vi "Add ECAT Slave from Config.vi"(8 "error in (no error)":errorcluster, 10 "Section Ptr":T4 format="%.0x", 11 "Slave":T1) -> (0 "error out":errorcluster)   [LabVIEW 2019, in "SEECD System Explorer.lvlib"]
uses:
  SEECD System Explorer.lvlib
  <vilib>/NI VeriStand/Custom Device API/Custom Device Item Ref.ctl
  Type Defs/Host - Slave.ctl
  Type Defs/Host - Module.ctl
  Type Defs/IOV Container Contents.ctl
  <vilib>/NI VeriStand/Custom Device API/Custom Device Channel.ctl
  <vilib>/NI VeriStand/Custom Device API/Custom Device Channel Type.ctl
  Includes/Modules.lvlibp/RSI Module/Slot Settings.ctl
  Includes/Modules.lvlibp/RSI Module/Module Models.ctl
  Shared/Globals/Scan Engine GUIDs.vi
  Shared/Globals/String Constants.vi
  Shared/Globals/Property Strings.vi
  <vilib>/NI VeriStand/Custom Device API/Set Item Property (String).vi
  Includes/Modules.lvlibp/RSI Module/Class Property Strings.vi
  Includes/Modules.lvlibp/RemIO Module/RemIO Module.lvclass
  Includes/Modules.lvlibp/RSI Module/RSI Module.lvclass
  <vilib>/NI VeriStand/Custom Device API/Custom Device API.lvlib
  Shared/SEECD Shared.lvlib
  Includes/Modules.lvlibp
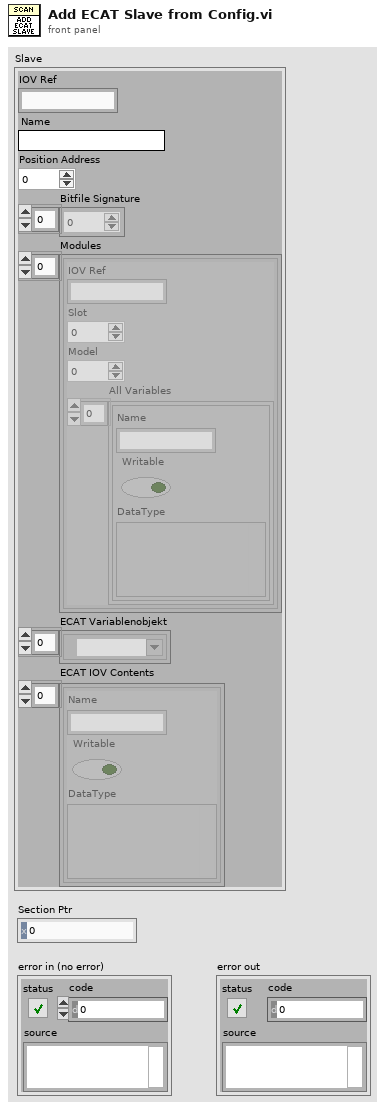
[diagram p1: front panel]
types:
  T1 = typedef "SEECD System Explorer.lvlib/Host - Slave.ctl" = cluster{"IOV Ref":string, "Name":string, "Position Address":u16, "Bitfile Signature":u8[], "Modules":T2[], "ECAT Variablenobjekt":refnum<k21>[], "ECAT IOV Contents":T3[]}
  T2 = typedef "SEECD System Explorer.lvlib/Host - Module.ctl" = cluster{"IOV Ref":string, "Slot":u32, "Model":u32, "All Variables":T3[]}
  T3 = typedef "SEECD System Explorer.lvlib/IOV Container Contents.ctl" = cluster{"Name":string, "Writable":bool, "DataType":variant}
  T4 = typedef "Custom Device API.lvlib/Custom Device Item Ref.ctl" = u64
  T5 = typedef "Custom Device API.lvlib/Custom Device Channel Type.ctl" = enum16{"Input", "Output"}
  T6 = typedef "Modules.lvlibp/RSI Module.lvclass/Slot Settings.ctl" = cluster{"Slot":u32, "EtherCAT?":bool}
  T7 = typedef "Modules.lvlibp/RSI Module.lvclass/Module Models.ctl" = enum16{"Empty", "NI 9201", "NI 9203", "NI 9205", "NI 9206", "NI 9207", "NI 9208", "NI 9209", "NI 9210", "NI 9211", "NI 9212", "NI 9213", "NI 9214", "NI 9215", "NI 9216", "NI 9217", "NI 9219", "NI 9220", "NI 9221", "NI 9222", "NI 9223", "NI 9224", "NI 9225", "NI 9226", "NI 9227", "NI 9228", "NI 9229", "NI 9233", "NI 9234", "NI 9235", "NI 9236", "NI 9237", "NI 9239", "NI 9242", "NI 9244", "NI 9253", "NI 9263", "NI 9264", "NI 9265", "NI 9266", "NI 9269", "NI 9344", "NI 9350", "NI 9375", "NI 9401", "NI 9402", "NI 9403", "NI 9411", "NI 9421", "NI 9422", "NI 9423", "NI 9425", "NI 9426", "NI 9435", "NI 9436", "NI 9437", "NI 9472", "NI 9474", "NI 9475", "NI 9476", "NI 9477", "NI 9478", "NI 9481", "NI 9482", "NI 9485"}
  T8 = typedef "Custom Device API.lvlib/Custom Device Channel.ctl" = cluster{"Type":T5, "Units":string, "Default Value":dbl, "Faultable":bool, "Scalable":bool}
  T9 = typedef "SEECD Shared.lvlib/ECAT Channel Data Type.ctl" = enum16{"Boolean", "Fixed Point", "Int8", "Int16", "Int32", "Int64", "U32 Bit Field", "UInt8", "UInt16", "UInt32", "UInt64", "Other", "DBL", "SGL"}
  T10 = typedef "Modules.lvlibp/Custom Device API.lvlib/Custom Device Item Ref.ctl" = u64
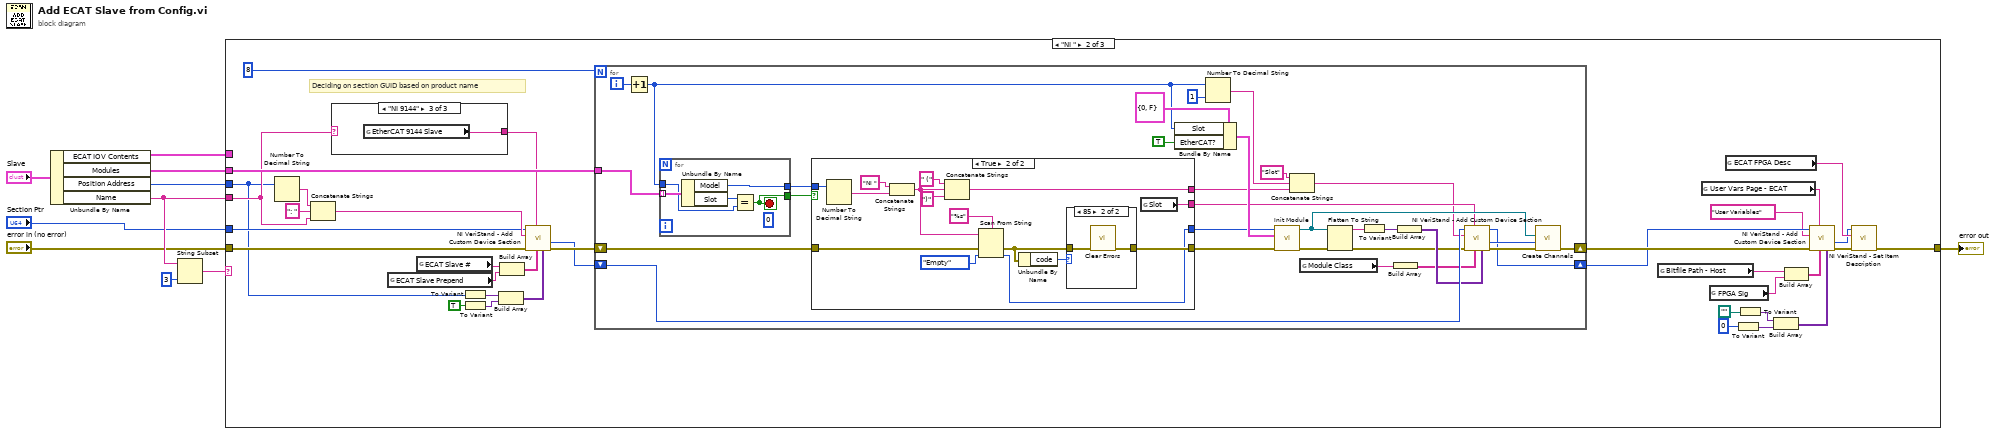
[diagram p0: block diagram]
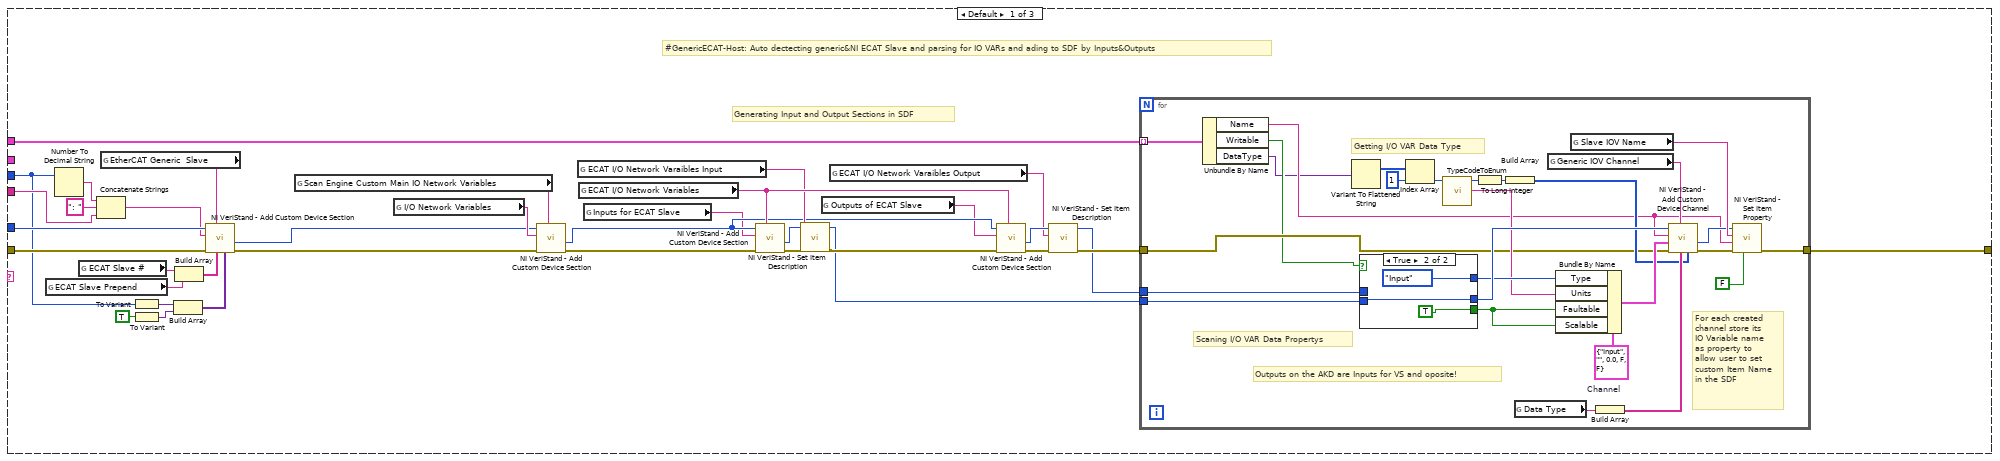
[diagram p2: hidden frame]
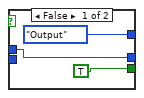
[diagram p3: hidden frame]
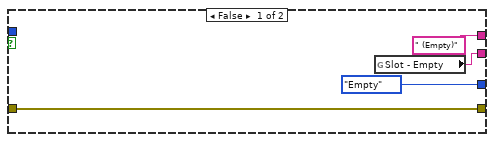
[diagram p4: hidden frame]
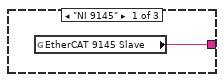
[diagram p6: hidden frame]
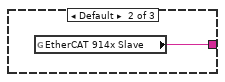
[diagram p7: hidden frame]
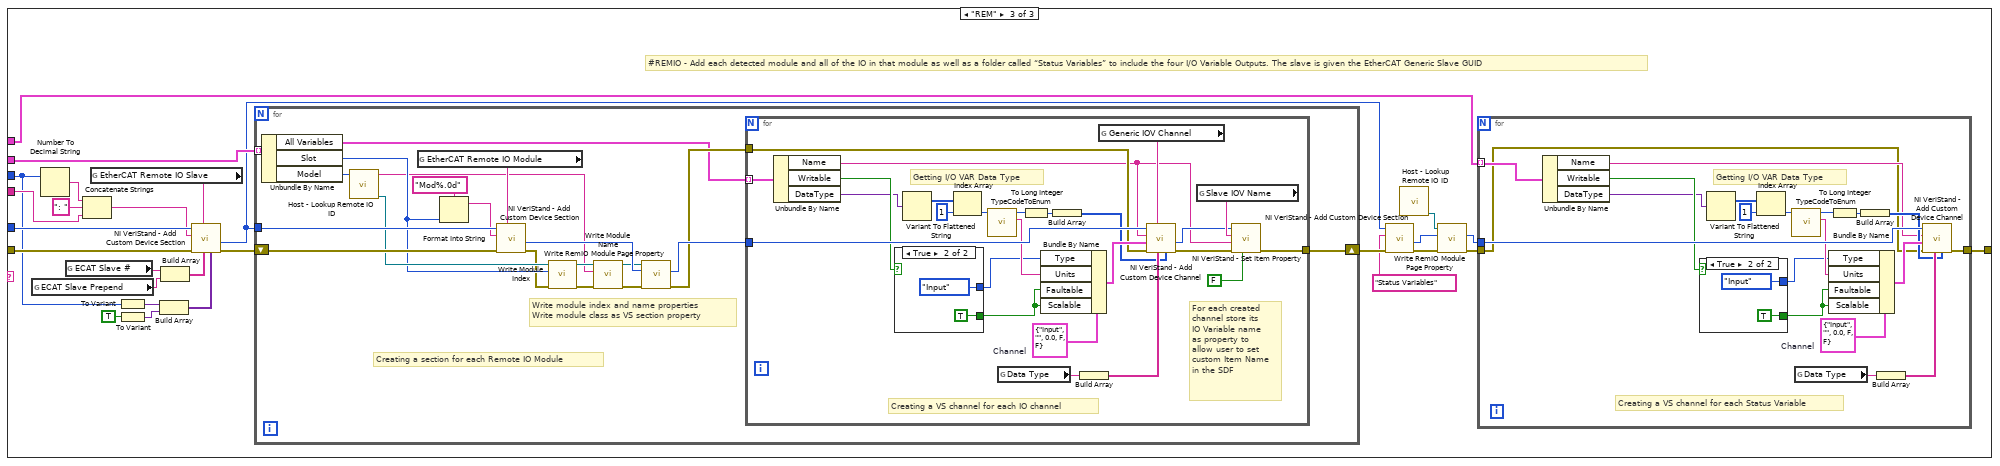
[diagram p8: hidden frame]
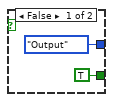
[diagram p9: hidden frame]
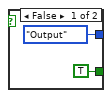
[diagram p10: hidden frame]
diagram:
  n1 = Unbundle By Name("Slave") -> ("ECAT IOV Contents"=w7:T3[], "Modules"=w4:T2[], "Position Address"=w9:u16, "Name"=w10:string)
  n2 = String Subset(string=w10, length (rest)=3 ("Länge (Rest)")) -> (substring=w8:string)  [unwired: 1 in]
  n3 = case shown="\"NI \"" w8 {
    tunnel: "error in (no error)" -> [w28 w98 w191]
    tunnel: w4 -> [_ w97 w200]
    tunnel: [w45 w96 w198] -> w5
    tunnel: w7 -> [w46 _ w197]
    tunnel: "Section Ptr" -> [w27 w83 w188]
    tunnel: w9 -> [w11 w80 w175]
    tunnel: w10 -> [w14 w82 w178]
    frame Default {
      # "#GenericECAT-Host: Auto dectecting generic&NI ECAT Slave and parsing for IO VARs and ading to SDF by Inputs&Outputs"
      # "Generating Input and Output Sections in SDF"
      n4 = global read "Property Strings.vi" "ECAT Slave Prepend"() -> (w18:string)
      n5 = Number To Decimal String(number=w11) -> (decimal integer string=w21:string)  [unwired: 1 in]
      n6 = global read "Property Strings.vi" "ECAT Slave #"() -> (w19:string)
      n7 = Concatenate Strings(w21, ": " ("string"), w14) -> (w23:string)
      n8 = global read "Scan Engine GUIDs.vi" "EtherCAT Generic  Slave"() -> (w24:string)
      n9 = To Variant(anything=w11) -> (Variant=w17:variant)
      n10 = To Variant(anything=TRUE) -> (Variant=w16:variant)
      n11 = Build Array(w17, w16) -> (w13:variant[])
      n12 = Build Array(w19, w18) -> (w20:string[])
      n13 = call <vilib>:"NI VeriStand - Add Custom Device Section.vi"("Property Values"=w13, "Property names"=w20, "GUID (Default Section)"=w24, "error in (no error)"=w28, "Section Name"=w23, "Parent Ref in"=w27) -> ("error out"=w25:errorcluster, "Section Ptr"=w26:T4)  [unwired: 2 in, 2 out]
      n14 = global read "Scan Engine GUIDs.vi" "Scan Engine Custom Main IO Network Variables"() -> (w38:string)
      n15 = global read "Property Strings.vi" "I/O Network Variables"() -> (w31:string)
      n16 = call <vilib>:"NI VeriStand - Add Custom Device Section.vi"("GUID (Default Section)"=w38, "error in (no error)"=w25, "Section Name"=w31, "Parent Ref in"=w26) -> ("error out"=w32:errorcluster, "Section Ptr"=w33:T4)  [unwired: 4 in, 2 out]
      n17 = global read "String Constants.vi" "ECAT I/O Network Varaibles Input"() -> (w34:string)
      n18 = global read "Scan Engine GUIDs.vi" "ECAT I/O Network Variables"() -> (w35:string)
      n19 = global read "Property Strings.vi" "Inputs for ECAT Slave"() -> (w30:string)
      n20 = call <vilib>:"NI VeriStand - Add Custom Device Section.vi"("GUID (Default Section)"=w35, "error in (no error)"=w32, "Section Name"=w30, "Parent Ref in"=w33) -> ("error out"=w44:errorcluster, "Section Ptr"=w37:T4)  [unwired: 4 in, 2 out]
      n21 = call <vilib>:"NI VeriStand - Set Item Description.vi"("error in (no error)"=w44, "Description"=w34, "Item Ref in"=w37) -> ("error out"=w43:errorcluster, "Item Ref out"=w42:T4)  [unwired: 6 in, 1 out]
      n22 = global read "Property Strings.vi" "Outputs of ECAT Slave"() -> (w29:string)
      n23 = global read "String Constants.vi" "ECAT I/O Network Varaibles Output"() -> (w12:string)
      n24 = call <vilib>:"NI VeriStand - Add Custom Device Section.vi"("GUID (Default Section)"=w35, "error in (no error)"=w43, "Section Name"=w29, "Parent Ref in"=w33) -> ("error out"=w41:errorcluster, "Section Ptr"=w36:T4)  [unwired: 4 in, 2 out]
      n25 = call <vilib>:"NI VeriStand - Set Item Description.vi"("error in (no error)"=w41, "Description"=w12, "Item Ref in"=w36) -> ("error out"=w40:errorcluster, "Item Ref out"=w39:T4)  [unwired: 6 in, 1 out]
      n26 = for {
        tunnel: w46 -> [w50] mode=indexing
        tunnel: [w55] -> w45
        tunnel: w40 -> [w51]
        tunnel: w39 -> [w68]
        tunnel: w42 -> [w66]
        w73 = T8 {"Type"=enum."Input", "Units"="", "Default Value"=0.0, "Faultable"=FALSE, "Scalable"=FALSE}  # Channel
        # "For each created channel store its IO Variable name as property to allow user to set custom Item Name in the SDF"
        # "Getting I/O VAR Data Type"
        # "Scaning I/O VAR Data Propertys"
        # "Outputs on the AKD are Inputs for VS and oposite!"
        n27 = Unbundle By Name(w50) -> ("Name"=w49:string, "Writable"=w48:bool, "DataType"=w47:variant)
        n28 = Variant To Flattened String(Variant=w47) -> (1:w70:i16[])  [unwired: 1 out]
        n29 = case shown="True" w48 {
          tunnel: [Custom_Device_Channel_Type."Output" ("Type") Custom_Device_Channel_Type."Input" ("Type")] -> w62
          tunnel: [w74 w77] -> w67
          tunnel: w68 -> [w74 _]
          tunnel: w66 -> [_ w77]
          tunnel: [TRUE TRUE] -> w65
          frame False {
          }
          frame True {
          }
        }
        n30 = Index Array(array=w70, index=1) -> (element=w60:i16)
        n31 = call "TypeCodeToEnum.vi"("Type Code (numbers in hexadecimal)"=w60) -> (2:"UDV Data Type"=w61:string, 3:"UDV Data Type"=w58:T9)  [unwired: 9 in]
        n32 = To Long Integer(number=w58) -> (32bit integer=w59:i32)
        n33 = Build Array(w59) -> (w63:i32[])
        n34 = global read "Property Strings.vi" "Data Type"() -> (w64:string)
        n35 = global read "Scan Engine GUIDs.vi" "Generic IOV Channel"() -> (w57:string)
        n36 = Bundle By Name(cluster=w73, "Type"=w62, "Units"=w61, "Faultable"=w65, "Scalable"=w65) -> (w72:T8)
        n37 = global read "Property Strings.vi" "Slave IOV Name"() -> (w53:string)
        n38 = Build Array(w64) -> (w71:string[])
        n39 = call <vilib>:"NI VeriStand - Add Custom Device Channel.vi"("Property Values"=w63, "Property names"=w71, "GUID (Default Channel)"=w57, "error in (no error)"=w51, "Channel"=w72, "Channel Name"=w49, "Parent Ref in"=w67) -> ("error out"=w56:errorcluster, "Channel Ref"=w52:T4)  [unwired: 1 in, 2 out]
        n40 = call-poly <vilib>:"NI VeriStand - Set Item Property.vi"("Binary String (T)"=FALSE, "error in (no error)"=w56, "Value"=w49, "Property Name"=w53, "Item Ref in"=w52) -> ("error out"=w55:errorcluster)  [unwired: 4 in, 2 out]
      }
    }
    frame "NI " {
      # "Deciding on section GUID based on product name"
      n41 = Number To Decimal String(number=w80) -> (decimal integer string=w94:string)  [unwired: 1 in]
      n42 = Concatenate Strings(w94, ": " ("string"), w82) -> (w92:string)
      n43 = case shown="\"NI 9144\"" w82 {
        tunnel: [w171 w172 w173] -> w81
        frame "NI 9145" {
          n44 = global read "Scan Engine GUIDs.vi" "EtherCAT 9145 Slave"() -> (w171:string)
        }
        frame Default {
          n45 = global read "Scan Engine GUIDs.vi" "EtherCAT 914x Slave"() -> (w172:string)
        }
        frame "NI 9144" {
          n46 = global read "Scan Engine GUIDs.vi" "EtherCAT 9144 Slave"() -> (w173:string)
        }
      }
      n47 = global read "Property Strings.vi" "ECAT Slave Prepend"() -> (w90:string)
      n48 = global read "Property Strings.vi" "ECAT Slave #"() -> (w89:string)
      n49 = To Variant(anything=w80) -> (Variant=w91:variant)
      n50 = To Variant(anything=TRUE) -> (Variant=w85:variant)
      n51 = Build Array(w91, w85) -> (w87:variant[])
      n52 = Build Array(w89, w90) -> (w88:string[])
      n53 = call <vilib>:"NI VeriStand - Add Custom Device Section.vi"("Property Values"=w87, "Property names"=w88, "GUID (Default Section)"=w81, "Section Name"=w92, "Parent Ref in"=w83) -> ("Section Ptr"=w84:T4)  [unwired: 3 in, 3 out]
      n54 = for {
        N: 8 -> [_]
        shift-right: [w117] -> w109
        shift-left: w98 -> [w123]
        shift-right: [w115] -> w108
        shift-left: w84 -> [w143]
        tunnel: w97 -> [w128]
        i -> [w140]
        n55 = Increment(x=w140) -> (x+1=w127:i32)
        n56 = for {
          tunnel: w128 -> [w170] mode=indexing
          tunnel: w127 -> [w168]
          tunnel: [w167] -> w126
          tunnel: [w166] -> w121
          stop <- w167 stop-if-true
          (unwired) u32 0 ("Model")
          n57 = Unbundle By Name(w170) -> ("Model"=w166:u32, "Slot"=w169:u32)
          n58 = Equal?(x=w169, y=w168) -> (x = y?=w167:bool)
        }
        n59 = case shown="True" w126 {
          tunnel: [" (Empty)" ("Section Name") w149] -> w125
          tunnel: [Module_Models."Empty" ("Module") w156] -> w124
          tunnel: w123 -> [w145 w157]
          tunnel: [w145 w158] -> w122
          tunnel: w121 -> [_ w155]
          tunnel: [w144 w148] -> w116
          frame False {
            n60 = global read "Scan Engine GUIDs.vi" "Slot - Empty"() -> (w144:string)
          }
          frame True {
            n61 = Number To Decimal String(number=w155) -> (decimal integer string=w154:string)  [unwired: 1 in]
            n62 = Concatenate Strings("NI " ("string"), w154) -> (w152:string)
            n63 = Concatenate Strings(" (" ("string"), w152, ")" ("string")) -> (w149:string)
            n64 = Scan From String(format string="%s", input string=w152, error in=w157, default 1=Module_Models."Empty" ("Module")) -> (error out=w159:errorcluster, output 1=w156:T7)  [unwired: 1 in, 2 out]
            n65 = Unbundle By Name(w159) -> ("code"=w160:i32)
            n66 = case shown="85" w160 {
              tunnel: [w163 w164] -> w158
              tunnel: w159 -> [w163 w165]
              frame 0, Default {
              }
              frame 85 {
                n67 = call <vilib>:"Clear Errors.vi"("error in (no error)"=w165) -> ("error out"=w164:errorcluster)  [unwired: 5 in, 1 out]
              }
            }
            n68 = global read "Scan Engine GUIDs.vi" "Slot"() -> (w148:string)
          }
        }
        n69 = Bundle By Name(cluster=T6 {"Slot"=0, "EtherCAT?"=FALSE} ("Slot Settings"), "Slot"=w127, "EtherCAT?"=TRUE) -> (w137:T6)
        n70 = Number To Decimal String(number=w127, width (-)=i16 1) -> (decimal integer string=w142:string)
        n71 = call "Init Module.vi"("error in (no error)"=w122, "Slot Settings"=w137, "Module Model"=w124) -> ("error out"=w132:errorcluster, "RSI Module out"=w118:refnum<class "RSI Module.lvclass">)  [unwired: 7 in]
        n72 = Concatenate Strings("Slot" ("string"), w142, w125) -> (w114:string)
        n73 = global read "Class Property Strings.vi" "Module Class"() -> (w130:string)
        n74 = Flatten To String(anything=w118, error in (no error)=w132) -> (data string=w133:string, error out=w131:errorcluster)  [unwired: 2 in, 1 out]
        n75 = To Variant(anything=w133) -> (Variant=w138:variant)
        n76 = Build Array(w130) -> (w134:string[])
        n77 = Build Array(w138) -> (w139:variant[])
        n78 = call <vilib>:"NI VeriStand - Add Custom Device Section.vi"("Property Values"=w139, "Property names"=w134, "GUID (Default Section)"=w116, "error in (no error)"=w131, "Section Name"=w114, "Parent Ref in"=w143) -> ("error out"=w119:errorcluster, "Section Ptr"=w120:T4, "Parent Ref out"=w115:T4)  [unwired: 2 in, 1 out]
        n79 = call-dynamic "Create Channels.vi"("error in (no error)"=w119, "RSI Module in"=w118, "Parent Ref in"=w120) -> ("error out"=w117:errorcluster)  [unwired: 6 in, 2 out]
      }
      n80 = global read "Property Strings.vi" "Bitfile Path - Host"() -> (w100:string)
      n81 = global read "Scan Engine GUIDs.vi" "User Vars Page - ECAT"() -> (w111:string)
      n82 = global read "Property Strings.vi" "FPGA Sig"() -> (w99:string)
      n83 = global read "String Constants.vi" "ECAT FPGA Desc"() -> (w110:string)
      n84 = To Variant(anything=u32 0 ("ModuleIdent (ECAT)")) -> (Variant=w101:variant)
      n85 = To Variant(anything=path "") -> (Variant=w102:variant)
      n86 = Build Array(w102, w101) -> (w112:variant[])
      n87 = Build Array(w100, w99) -> (w113:string[])
      n88 = call <vilib>:"NI VeriStand - Add Custom Device Section.vi"("Property Values"=w112, "Property names"=w113, "GUID (Default Section)"=w111, "error in (no error)"=w109, "Section Name"="User Variables", "Parent Ref in"=w108) -> ("error out"=w105:errorcluster, "Section Ptr"=w106:T4)  [unwired: 2 in, 2 out]
      n89 = call <vilib>:"NI VeriStand - Set Item Description.vi"("error in (no error)"=w105, "Description"=w110, "Item Ref in"=w106) -> ("error out"=w96:errorcluster)  [unwired: 6 in, 2 out]
    }
    frame "REM" {
      # "#REMIO - Add each detected module and all of the IO in that module as well as a folder called “Status Variables” to include the four I/O Variable Outputs. The slave is given the EtherCAT Generic Slave GUID"
      n90 = global read "Property Strings.vi" "ECAT Slave Prepend"() -> (w182:string)
      n91 = Number To Decimal String(number=w175) -> (decimal integer string=w186:string)  [unwired: 1 in]
      n92 = global read "Property Strings.vi" "ECAT Slave #"() -> (w181:string)
      n93 = Concatenate Strings(w186, ": " ("string"), w178) -> (w184:string)
      n94 = global read "Scan Engine GUIDs.vi" "EtherCAT Remote IO Slave"() -> (w187:string)
      n95 = To Variant(anything=w175) -> (Variant=w183:variant)
      n96 = To Variant(anything=TRUE) -> (Variant=w176:variant)
      n97 = Build Array(w183, w176) -> (w179:variant[])
      n98 = Build Array(w181, w182) -> (w180:string[])
      n99 = call <vilib>:"NI VeriStand - Add Custom Device Section.vi"("Property Values"=w179, "Property names"=w180, "GUID (Default Section)"=w187, "error in (no error)"=w191, "Section Name"=w184, "Parent Ref in"=w188) -> ("error out"=w190:errorcluster, "Section Ptr"=w189:T4)  [unwired: 2 in, 2 out]
      n100 = for {
        shift-right: [w217] -> w199
        shift-left: w190 -> [w220]
        tunnel: w189 -> [w219]
        tunnel: w200 -> [w218] mode=indexing
        # "Write module index and name properties\nWrite module class as VS section property"
        # "Creating a section for each Remote IO Module"
        n101 = Unbundle By Name(w218) -> ("All Variables"=w201:T3[], "Slot"=w214:u32, "Model"=w216:u32)
        n102 = call "Host - Lookup Remote IO ID.vi"("Module ID"=w216) -> ("RemIO Module Out"=w215:refnum<class "RemIO Module.lvclass">, "Module Name"=w203:string)  [unwired: 9 in]
        n103 = global read "Scan Engine GUIDs.vi" "EtherCAT Remote IO Module"() -> (w213:string)
        n104 = Format Into String(format string="Mod%.0d", w214) -> (resulting string=w209:string)  [unwired: 2 in, 1 out]
        n105 = call <vilib>:"NI VeriStand - Add Custom Device Section.vi"("GUID (Default Section)"=w213, "error in (no error)"=w220, "Section Name"=w209, "Parent Ref in"=w219) -> ("error out"=w211:errorcluster, "Section Ptr"=w212:T4)  [unwired: 4 in, 2 out]
        n106 = call-dynamic "Write Module Index.vi"("error in (no error)"=w211, "Module Index"=w214, "RemIO Module in"=w215) -> ("error out"=w206:errorcluster, "RemIO Module out"=w207:refnum<class "RemIO Module.lvclass">)  [unwired: 7 in]
        n107 = call-dynamic "Write Module Name.vi"("error in (no error)"=w206, "Module Name"=w203, "RemIO Module in"=w207) -> ("error out"=w205:errorcluster, "RemIO Module out"=w204:refnum<class "RemIO Module.lvclass">)  [unwired: 7 in]
        n108 = call "Write RemIO Module Page Property.vi"("error in (no error)"=w205, "Node Ptr In"=w212, "RemIO Module"=w204) -> ("error out"=w202:errorcluster, "Node Ptr Out"=w210:T10)  [unwired: 6 in, 1 out]
        n109 = for {
          tunnel: w210 -> [w245]
          tunnel: [w230] -> w217
          tunnel: w202 -> [w225]
          tunnel: w201 -> [w224] mode=indexing
          w244 = T8 {"Type"=enum."Input", "Units"="", "Default Value"=0.0, "Faultable"=FALSE, "Scalable"=FALSE}  # Channel
          # "For each created channel store its IO Variable name as property to allow user to set custom Item Name in the SDF"
          # "Creating a VS channel for each IO channel"
          # "Getting I/O VAR Data Type"
          n110 = Unbundle By Name(w224) -> ("Name"=w223:string, "Writable"=w222:bool, "DataType"=w221:variant)
          n111 = case shown="True" w222 {
            tunnel: [TRUE TRUE] -> w243
            tunnel: [Custom_Device_Channel_Type."Output" ("Type") Custom_Device_Channel_Type."Input" ("Type")] -> w233
            frame False {
            }
            frame True {
            }
          }
          n112 = Variant To Flattened String(Variant=w221) -> (1:w240:i16[])  [unwired: 1 out]
          n113 = Index Array(array=w240, index=1) -> (element=w242:i16)
          n114 = call "TypeCodeToEnum.vi"("Type Code (numbers in hexadecimal)"=w242) -> (2:"UDV Data Type"=w239:string, 3:"UDV Data Type"=w237:T9)  [unwired: 9 in]
          n115 = global read "Property Strings.vi" "Data Type"() -> (w236:string)
          n116 = To Long Integer(number=w237) -> (32bit integer=w232:i32)
          n117 = Bundle By Name(cluster=w244, "Type"=w233, "Units"=w239, "Faultable"=w243, "Scalable"=w243) -> (w238:T8)
          n118 = Build Array(w232) -> (w234:i32[])
          n119 = Build Array(w236) -> (w235:string[])
          n120 = global read "Scan Engine GUIDs.vi" "Generic IOV Channel"() -> (w228:string)
          n121 = call <vilib>:"NI VeriStand - Add Custom Device Channel.vi"("Property Values"=w234, "Property names"=w235, "GUID (Default Channel)"=w228, "error in (no error)"=w225, "Channel"=w238, "Channel Name"=w223, "Parent Ref in"=w245) -> ("error out"=w231:errorcluster, "Channel Ref"=w226:T4)  [unwired: 1 in, 2 out]
          n122 = global read "Property Strings.vi" "Slave IOV Name"() -> (w229:string)
          n123 = call-poly <vilib>:"NI VeriStand - Set Item Property.vi"("Binary String (T)"=FALSE, "error in (no error)"=w231, "Value"=w223, "Property Name"=w229, "Item Ref in"=w226) -> ("error out"=w230:errorcluster)  [unwired: 4 in, 2 out]
        }
      }
      n124 = call <vilib>:"NI VeriStand - Add Custom Device Section.vi"("error in (no error)"=w199, "Section Name"="Status Variables", "Parent Ref in"=w189) -> ("error out"=w196:errorcluster, "Section Ptr"=w194:T4)  [unwired: 5 in, 2 out]
      n125 = call "Host - Lookup Remote IO ID.vi"() -> ("RemIO Module Out"=w192:refnum<class "RemIO Module.lvclass">)  [unwired: 10 in, 1 out]
      n126 = call "Write RemIO Module Page Property.vi"("error in (no error)"=w196, "Node Ptr In"=w194, "RemIO Module"=w192) -> ("error out"=w195:errorcluster, "Node Ptr Out"=w193:T10)  [unwired: 6 in, 1 out]
      n127 = for {
        tunnel: w197 -> [w254] mode=indexing
        tunnel: w193 -> [w269]
        tunnel: [w256] -> w198
        tunnel: w195 -> [w250]
        w268 = T8 {"Type"=enum."Input", "Units"="", "Default Value"=0.0, "Faultable"=FALSE, "Scalable"=FALSE}  # Channel
        # "Creating a VS channel for each Status Variable"
        # "Getting I/O VAR Data Type"
        n128 = Unbundle By Name(w254) -> ("Name"=w253:string, "Writable"=w252:bool, "DataType"=w251:variant)
        n129 = case shown="True" w252 {
          tunnel: [Custom_Device_Channel_Type."Output" ("Type") Custom_Device_Channel_Type."Input" ("Type")] -> w255
          tunnel: [TRUE TRUE] -> w267
          frame False {
          }
          frame True {
          }
        }
        n130 = Variant To Flattened String(Variant=w251) -> (1:w264:i16[])  [unwired: 1 out]
        n131 = Index Array(array=w264, index=1) -> (element=w266:i16)
        n132 = call "TypeCodeToEnum.vi"("Type Code (numbers in hexadecimal)"=w266) -> (2:"UDV Data Type"=w263:string, 3:"UDV Data Type"=w258:T9)  [unwired: 9 in]
        n133 = global read "Property Strings.vi" "Data Type"() -> (w261:string)
        n134 = Bundle By Name(cluster=w268, "Type"=w255, "Units"=w263, "Faultable"=w267, "Scalable"=w267) -> (w262:T8)
        n135 = To Long Integer(number=w258) -> (32bit integer=w259:i32)
        n136 = Build Array(w259) -> (w257:i32[])
        n137 = Build Array(w261) -> (w260:string[])
        n138 = call <vilib>:"NI VeriStand - Add Custom Device Channel.vi"("Property Values"=w257, "Property names"=w260, "error in (no error)"=w250, "Channel"=w262, "Channel Name"=w253, "Parent Ref in"=w269) -> ("error out"=w256:errorcluster)  [unwired: 2 in, 3 out]
      }
    }
  }
  "error out" <- w5
